vi "Browse_Disk_Client.vi"(1 "Start Path":path=path "C:/EnFlo_Data_Temp") -> (0 "Folder to Pull from Server":path)   [LabVIEW 2013]
uses:
  Anemometry/Anemometry Sub Vis/Globals/Preference_global.vi
panel:
  in  "OK Button":bool
  out "Folder":string[](array[string])
  in  "Depth":i32=1 min=1 max=7
  in  "Level 7":u16(ring)
  in  "Level 6":u16(ring)
  in  "Level 5":u16(ring) items=["01-2013", "02-2013", "03-2013", "04-2013", "05-2013", "06-2013", "07-2013", "09-2013", "10-2013"]
  in  "Level 1":u16(ring) items=["1997", "1998", "1999", "2000", "2001", "2002", "2003", "2004", "2005", "2006", "2007", "2008", "2009", "2010", "2011", "2012", "2013", "Archive", "Network Trash Folder", "Preferences", "Temporary Items"]
  in  "Level 4":u16(ring) items=["Calibrations", "Commands", "Logs", "Pictures", "Preferences", "Raw_Calibrations", "Raw_Measurements", "Results", "Results_Post_Processed", "Videos"]
  in  "Level 3":u16(ring) items=["Aidan_Brocklehurst", "fred", "Joe_Batten", "Paul_Hayden", "Robert_Spencer", "Shanying_Zhang", "Toblerone", "Tom_Farr", "Ugur_Ecin", "William_Wou"]
  out "Files":string[](array[string])
  in  "Level 2":u16(ring) items=["A_Tunnel", "ADAM_Server", "Aero_Server", "Aero_Tunnel", "B_Tunnel", "Captured Files", "D_Tunnel", "EnFlo_Tunnel", "Fruit_Rig", "Soil_Rig", "Tank"]
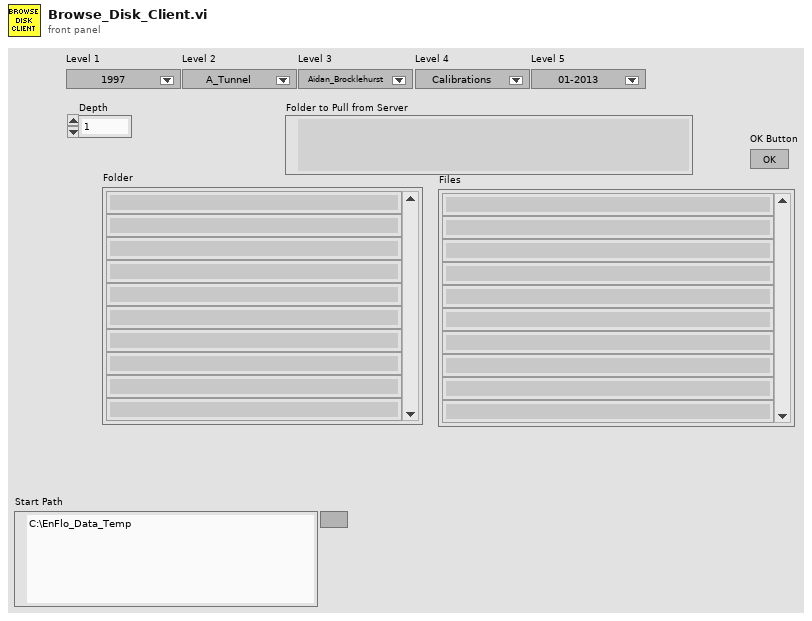
[diagram p1: front panel]
types:
  T1 = cluster{"folder names":string[], "filenames":string[]}
  T2 = cluster{"folder names":string[], "filenames":string[]}[]
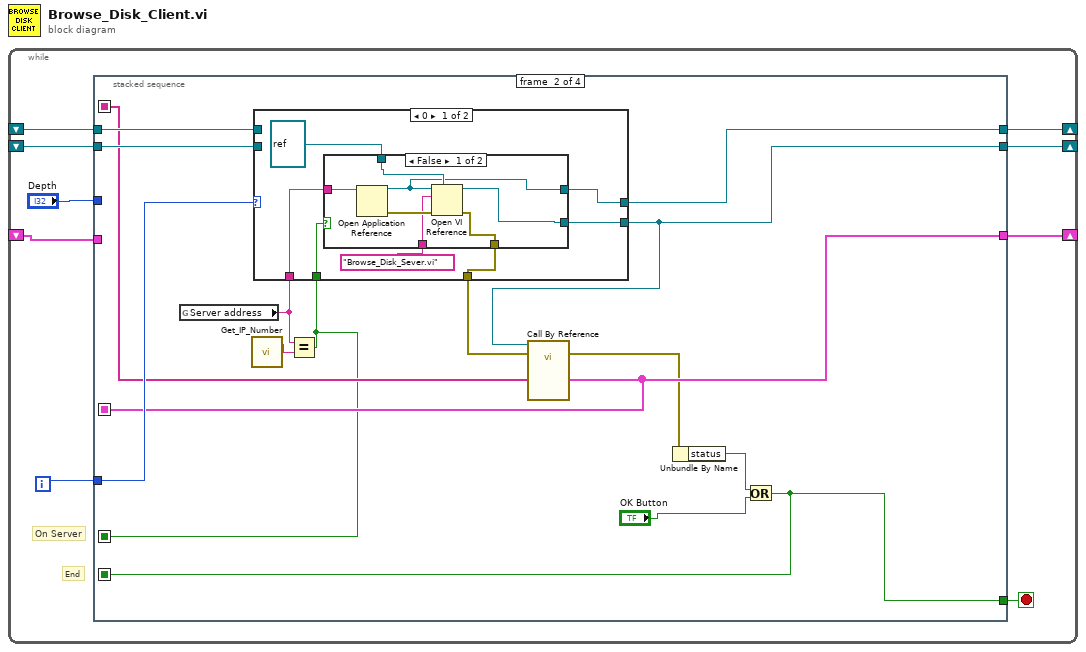
[diagram p0: block diagram]
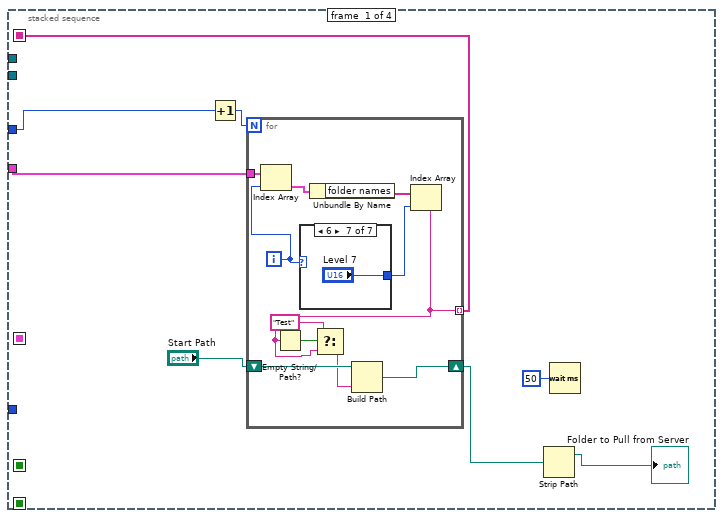
[diagram p2: hidden frame]
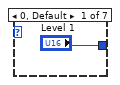
[diagram p3: hidden frame]
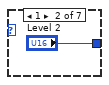
[diagram p4: hidden frame]
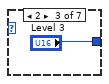
[diagram p5: hidden frame]
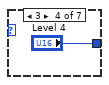
[diagram p6: hidden frame]
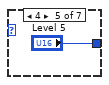
[diagram p7: hidden frame]
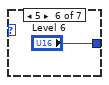
[diagram p8: hidden frame]
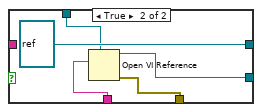
[diagram p9: hidden frame]
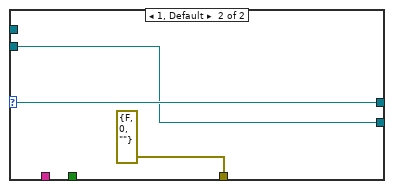
[diagram p10: hidden frame]
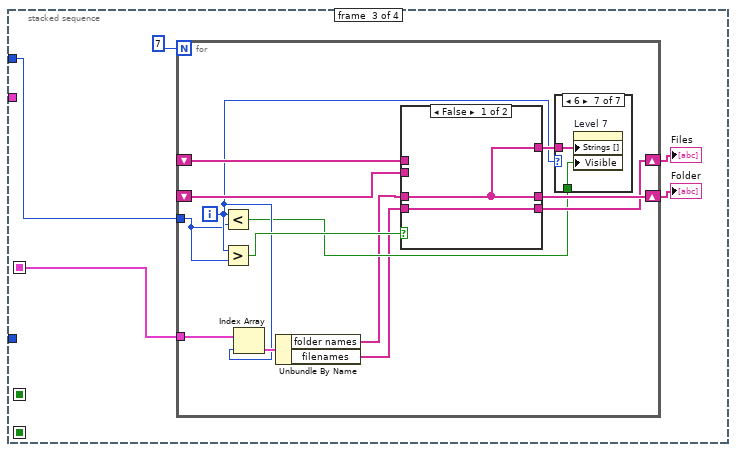
[diagram p11: hidden frame]
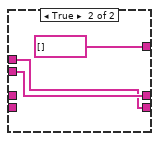
[diagram p12: hidden frame]
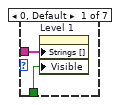
[diagram p13: hidden frame]
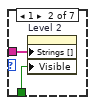
[diagram p14: hidden frame]
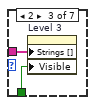
[diagram p15: hidden frame]
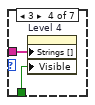
[diagram p16: hidden frame]
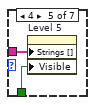
[diagram p17: hidden frame]
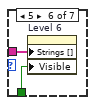
[diagram p18: hidden frame]
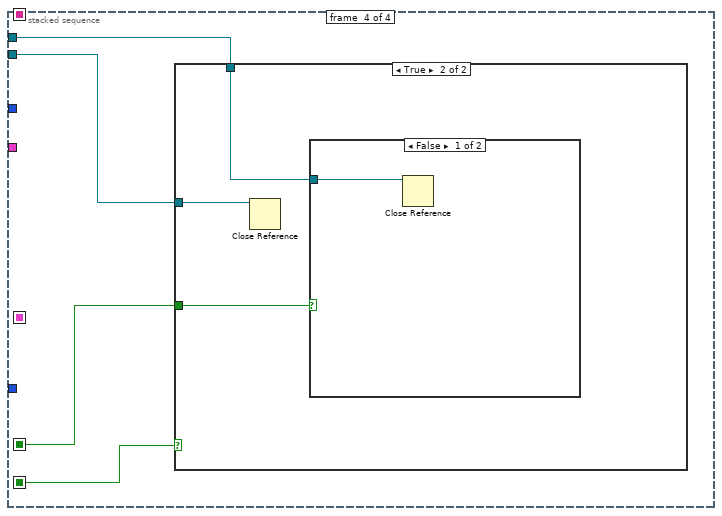
[diagram p19: hidden frame]
diagram:
  n1 = while {
    shift-right: [w7] -> _
    shift-left: _ -> [w9]
    shift-right: [w5] -> _
    shift-left: _ -> [w4]
    shift-right: [w2] -> _
    shift-left: _ -> [w3]
    i -> [w6]
    stop <- w1 stop-if-true
    # "End"
    # "On Server"
    n2 = stacked-sequence {
      seq-local: [w10 _ _ _] -> [_ w43 _ _]
      seq-local: [_ w42 _ _] -> [_ _ w73 _]
      seq-local: [_ w38 _ _] -> [_ _ _ w113]
      seq-local: [_ w37 _ _] -> [_ _ _ w111]
      tunnel: w9 -> [w16 _ _ _]
      tunnel: "Depth" -> [w14 _ w74 _]
      tunnel: [_ w42 _ _] -> w7
      tunnel: w6 -> [_ w50 _ _]
      tunnel: [_ w49 _ _] -> w5
      tunnel: w4 -> [_ w48 _ w110]
      tunnel: w3 -> [_ w45 _ w112]
      tunnel: [_ w44 _ _] -> w2
      tunnel: [_ w38 _ _] -> w1
      frame #0 {
        n3 = Increment(x=w14) -> (x+1=w15:i32)
        n4 = for {
          N: w15 -> [_]
          tunnel: w16 -> [w26]
          shift-right: [w22] -> w12
          shift-left: "Start Path" -> [w23]
          tunnel: [w20] -> w10 mode=indexing
          i -> [w25]
          n5 = Index Array(array=w26, index=w25) -> (element=w24:T1)
          n6 = case shown="6" w25 {
            tunnel: ["Level 1" "Level 2" "Level 3" "Level 4" "Level 5" "Level 6" "Level 7"] -> w27
            frame 0, Default {
            }
            frame 1 {
            }
            frame 2 {
            }
            frame 3 {
            }
            frame 4 {
            }
            frame 5 {
            }
            frame 6 {
            }
          }
          n7 = Unbundle By Name(w24) -> ("folder names"=w28:string[])
          n8 = Index Array(array=w28, index=w27) -> (element=w20:string)
          n9 = Empty String/Path?(string/path=w20) -> (empty?=w21:bool)
          n10 = Select(t="Test", s=w21, f=w20) -> (s? t:f=w19:string)
          n11 = Build Path(base path=w23, name or relative path=w19) -> (appended path=w22:path)
        }
        n12 = Strip Path(path=w12) -> (stripped path=→"Folder to Pull from Server":path)  [unwired: 1 out]
        n13 = Wait (ms)(milliseconds to wait=u32 50) -> ()  [unwired: 1 out]
      }
      frame #1 {
        n14 = global read "Preference_global.vi" "Server address"() -> (w46:string)
        n15 = call "Get_IP_Number.vi"() -> ("IP Number"=w47:string)  [unwired: 1 out]
        n16 = Equal?(x=w46, y=w47) -> (x = y?=w37:bool)
        n17 = case shown="0" w50 {
          tunnel: [w57 w72] -> w49
          tunnel: w48 -> [_ w72]
          tunnel: w46 -> [w56 _]
          tunnel: w37 -> [w55 _]
          tunnel: [w53 w71] -> w44
          tunnel: w45 -> [_ w71]
          tunnel: [w51 errorcluster {"status"=FALSE, "code"=0, "source"=""} ("error out")] -> w41
          frame 0 {
            n18 = case shown="False" w55 {
              tunnel: [w59 refnum<vi> refnum ("application reference (local)")] -> w57
              tunnel: w56 -> [w64 _]
              tunnel: "Browse_Disk_Sever.vi" -> [w62 w68]
              tunnel: [w60 w67] -> w53
              tunnel: refnum<vi> refnum ("Scout Server") -> [w61 w66]
              tunnel: [w58 w65] -> w51
              frame False {
                n19 = Open Application Reference(11:w64) -> (0:w63:errorcluster, 3:w59:refnum<vi>)  [unwired: 2 in, 1 out]
                n20 = Open VI Reference(type specifier VI Refnum (for type only)=w61, application reference (local)=w59, vi path=w62, error in (no error)=w63) -> (vi reference=w60:refnum<vi>, error out=w58:errorcluster)  [unwired: 2 out]
              }
              frame True {
                n21 = Open VI Reference(type specifier VI Refnum (for type only)=w66, vi path=w68) -> (vi reference=w67:refnum<vi>, error out=w65:errorcluster)  [unwired: 2 in, 2 out]
              }
            }
          }
          frame 1, Default {
          }
        }
        n22 = call-by-ref "?"(reference=w44, error in=w41, "Folder Hierarchy"=w43) -> (error out=w40:errorcluster, "Folders and files"=w42:T2)  [unwired: 1 out]
        n23 = Unbundle By Name(w40) -> ("status"=w39:bool)
        n24 = Or(x=w39, y="OK Button") -> (x .or. y?=w38:bool)
      }
      frame #2 {
        n25 = for {
          N: 7 -> [_]
          tunnel: w73 -> [w90]
          tunnel: w74 -> [w81]
          shift-right: [w87] -> w76
          shift-left: _ -> [w85]
          shift-right: [w86] -> w75
          shift-left: _ -> [w84]
          i -> [w82]
          n26 = Less?(x=w82, y=w81) -> (x < y?=w80:bool)
          n27 = Greater?(x=w82, y=w81) -> (0:w83:bool)
          n28 = Index Array(array=w90, index=w82) -> (element=w89:T1)
          n29 = Unbundle By Name(w89) -> ("folder names"=w79:string[], "filenames"=w78:string[])
          n30 = case shown="False" w83 {
            tunnel: [w91 string[] [] ("folder names")] -> w88
            tunnel: w79 -> [w91 _]
            tunnel: [w91 w94] -> w87
            tunnel: w78 -> [w92 _]
            tunnel: [w92 w93] -> w86
            tunnel: w85 -> [_ w94]
            tunnel: w84 -> [_ w93]
            frame False {
            }
            frame True {
            }
          }
          n31 = case shown="6" w82 {
            tunnel: w88 -> [w97 w99 w101 w103 w105 w107 w109]
            tunnel: w80 -> [w96 w98 w100 w102 w104 w106 w108]
            frame 0, Default {
              n32 = property on="Level 1" class="Ring (strict)"("Strings []"=w97, "Visible"=w96) -> ()  [unwired: 2 in, 2 out]
            }
            frame 1 {
              n33 = property on="Level 2" class="Ring (strict)"("Strings []"=w99, "Visible"=w98) -> ()  [unwired: 2 in, 2 out]
            }
            frame 2 {
              n34 = property on="Level 3" class="Ring (strict)"("Strings []"=w101, "Visible"=w100) -> ()  [unwired: 2 in, 2 out]
            }
            frame 3 {
              n35 = property on="Level 4" class="Ring (strict)"("Strings []"=w103, "Visible"=w102) -> ()  [unwired: 2 in, 2 out]
            }
            frame 4 {
              n36 = property on="Level 5" class="Ring (strict)"("Strings []"=w105, "Visible"=w104) -> ()  [unwired: 2 in, 2 out]
            }
            frame 5 {
              n37 = property on="Level 6" class="Ring (strict)"("Strings []"=w107, "Visible"=w106) -> ()  [unwired: 2 in, 2 out]
            }
            frame 6 {
              n38 = property on="Level 7" class="Ring (strict)"("Strings []"=w109, "Visible"=w108) -> ()  [unwired: 2 in, 2 out]
            }
          }
        }
        "Files" <- w75
        "Folder" <- w76
      }
      frame #3 {
        n39 = case shown="True" w113 {
          tunnel: w112 -> [_ w116]
          tunnel: w111 -> [_ w115]
          tunnel: w110 -> [_ w114]
          frame False {
          }
          frame True {
            n40 = Close Reference(reference=w116) -> ()  [unwired: 1 in, 1 out]
            n41 = case shown="False" w115 {
              tunnel: w114 -> [w117 _]
              frame False {
                n42 = Close Reference(reference=w117) -> ()  [unwired: 1 in, 1 out]
              }
              frame True {
              }
            }
          }
        }
      }
    }
  }
